vi "item sink unknown.vi"(11 "Items in":u32[](array[numeric])) -> (2 "Items out":u32[](array[numeric]))   [LabVIEW 2025]
panel:
  out "zeros":u32
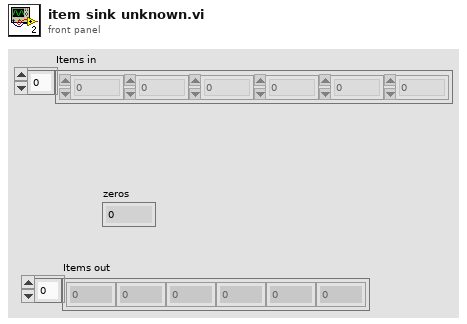
[diagram p1: front panel]
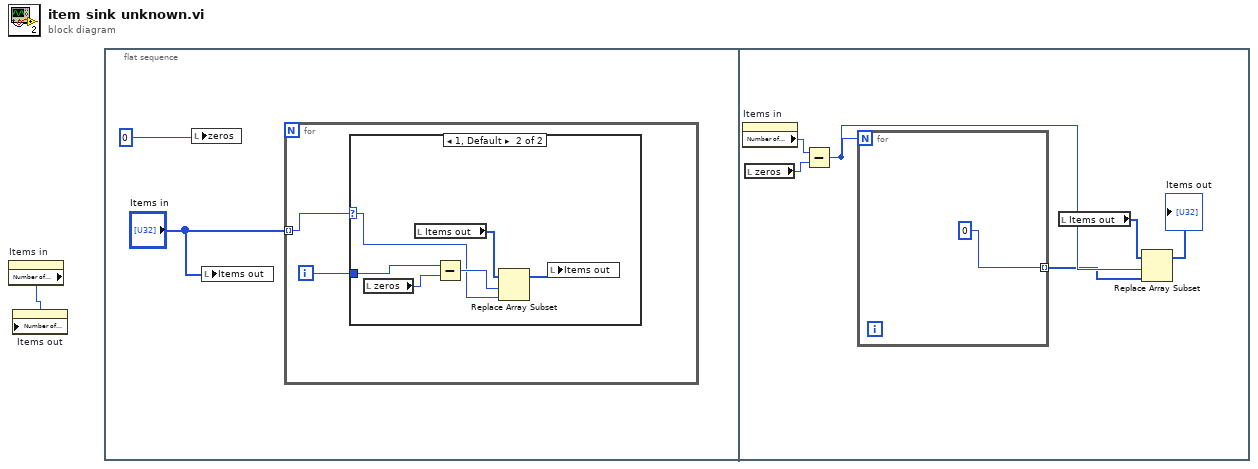
[diagram p0: block diagram]
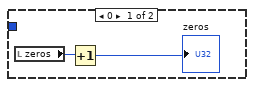
[diagram p2: hidden frame]
diagram:
  n1 = property on="Items in" class="Arr (strict)"() -> ("Number of Columns"=w1:u32)  [unwired: 2 in, 2 out]
  n2 = property on="Items out" class="Arr (strict)"("Number of Columns"=w1) -> ()  [unwired: 2 in, 2 out]
  n3 = flat-sequence {
    frame #0 {
      n4 = local write "zeros"(u32 0) -> ()
      n5 = local write "Items out"("Items in") -> ()
      n6 = for {
        tunnel: "Items in" -> [w5] mode=indexing
        i -> [w4]
        n7 = case shown="1, Default" w5 {
          selector: w5 -> [_ w8]
          tunnel: w4 -> [_ w13]
          frame 0 {
            n8 = local read "zeros"() -> (w7:u32)
            n9 = Increment(x=w7) -> (x+1=→"zeros":u32)
          }
          frame 1, Default {
            n10 = local read "zeros"() -> (w12:u32)
            n11 = local read "Items out"() -> (w9:u32[])
            n12 = Subtract(x=w13, y=w12) -> (x-y=w11:u32)
            n13 = Replace Array Subset(array=w9, new element=w8, index=w11) -> (w10:u32[])
            n14 = local write "Items out"(w10) -> ()
          }
        }
      }
    }
    frame #1 {
      n15 = property on="Items in" class="Arr (strict)"() -> ("Number of Columns"=w19:u32)  [unwired: 2 in, 2 out]
      n16 = local read "zeros"() -> (w18:u32)
      n17 = Subtract(x=w19, y=w18) -> (x-y=w17:u32)
      n18 = for {
        N: w17 -> [_]
        tunnel: [u32 0] -> w16 mode=indexing
      }
      n19 = local read "Items out"() -> (w15:u32[])
      n20 = Replace Array Subset(array=w15, new element=w16, index=w17) -> (→"Items out":u32[])
    }
  }
